vi "parse_tree.vi"() -> ()   [LabVIEW 2021]
uses:
  <vilib>/National Instruments/Tree Map/Tree Map.lvlib
panel:
  out "Pretty XML":string
  in  "Expression":string="(((1+2)*3)/(3+9))"
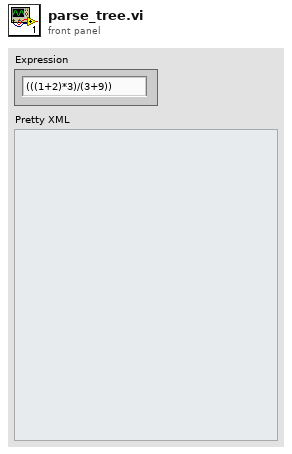
[diagram p1: front panel]
types:
  T1 = typedef "Tree Map.lvlib/Tree Map Data.ctl" = map{string, cluster{"Child Paths Set":set{string}, "Name":string, "Data":string, "Attributes":map{string, string}}}
  T2 = cluster{"Child Paths Set":set{string}, "Name":string, "Data":string, "Attributes":map{string, string}}
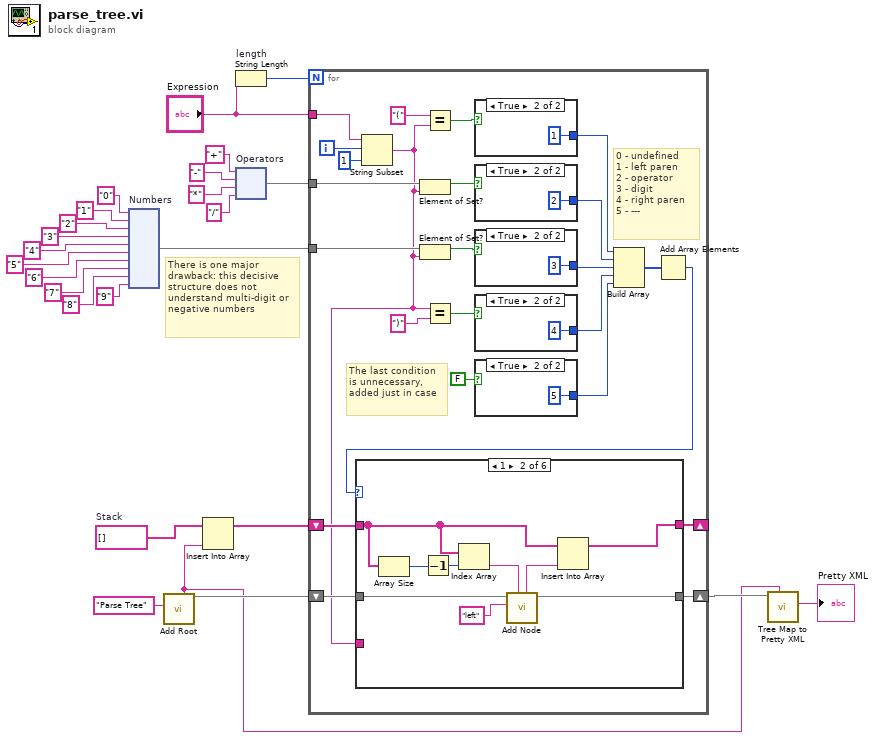
[diagram p0: block diagram]
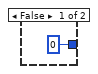
[diagram p2: hidden frame]
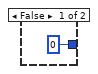
[diagram p3: hidden frame]
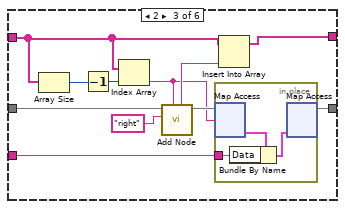
[diagram p5: hidden frame]
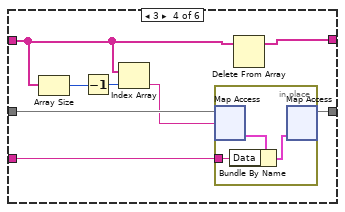
[diagram p6: hidden frame]
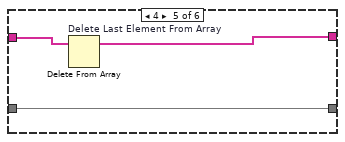
[diagram p7: hidden frame]
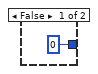
[diagram p9: hidden frame]
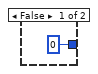
[diagram p10: hidden frame]
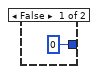
[diagram p11: hidden frame]
diagram:
  w6 = string[] []  # Stack
  # "There is one major drawback: this decisive structure does not understand multi-digit or negative numbers"
  n1 = node "Numbers"("0" ("element"), "1" ("element"), "2" ("element"), "3" ("element"), "4" ("element"), "5" ("element"), "6" ("element"), "7" ("element"), "8" ("element"), "9" ("element")) -> (w8:set{string})
  n2 = call <vilib>:"Add Root.vi"("New Root Name"="Parse Tree") -> ("Tree Map Out"=w3:T1, "Root Path"=w1:string)  [unwired: 9 in]
  n3 = Insert Into Array "Insert Into Array"(array=w6, new element=w1) -> (w5:string[])  [unwired: 1 in]
  n4 = String Length "length"(string="Expression") -> (length=w21:i32)
  n5 = node "Operators"("+" ("element"), "-" ("element"), "*" ("element"), "/" ("element")) -> (w9:set{string})
  n6 = for {
    N: w21 -> [_]
    tunnel: "Expression" -> [w49]
    tunnel: w9 -> [w45]
    tunnel: w8 -> [w43]
    shift-right: [w37] -> w2
    shift-left: w3 -> [w40]
    shift-right: [w38] -> _
    shift-left: w5 -> [w39]
    i -> [w48]
    # "The last condition is unnecessary, added just in case"
    # "0 - undefined\n1 - left paren\n2 - operator\n3 - digit\n4 - right paren\n5 - ---"
    n7 = String Subset(string=w49, offset (0)=w48, length (rest)=1 ("length (rest)")) -> (substring=w26:string)
    n8 = Element of Set?(10:w26, 11:w45) -> (3:w46:bool)
    n9 = Element of Set?(10:w26, 11:w43) -> (3:w44:bool)
    n10 = Equal?(x="(", y=w26) -> (x = y?=w30:bool)
    n11 = Equal?(x=w26, y=")" ("x")) -> (x = y?=w28:bool)
    n12 = case shown="True" w30 {
      tunnel: [0 1] -> w35
      frame False {
      }
      frame True {
      }
    }
    n13 = case shown="True" w46 {
      tunnel: [0 2] -> w32
      frame False {
      }
      frame True {
      }
    }
    n14 = case shown="True" w44 {
      tunnel: [0 3] -> w36
      frame False {
      }
      frame True {
      }
    }
    n15 = case shown="True" w28 {
      tunnel: [0 4] -> w33
      frame False {
      }
      frame True {
      }
    }
    n16 = case shown="True" FALSE {
      tunnel: [0 5] -> w34
      frame False {
      }
      frame True {
      }
    }
    n17 = Build Array(w35, w32, w36, w33, w34) -> (w42:i32[])
    n18 = Add Array Elements(numeric array=w42) -> (sum=w41:i32)
    n19 = case shown="1" w41 {
      tunnel: w40 -> [w54 w64 w72 w85 w92 w93]
      tunnel: w39 -> [w55 w59 w69 w80 w91 w94]
      tunnel: [w55 w61 w67 w79 w90 w94] -> w38
      tunnel: [w54 w60 w75 w86 w92 w93] -> w37
      tunnel: w26 -> [_ _ w65 w81 _ _]
      frame 0, Default {
      }
      frame 1 {
        n20 = Array Size(array=w59) -> (size(s)=w58:i32)
        n21 = Decrement(x=w58) -> (x-1=w57:i32)
        n22 = Index Array "Index Array"(array=w59, index=w57) -> (element=w62:string)
        n23 = call <vilib>:"Add Node.vi"("Parent Path"=w62, "New Node Name"="left", "Tree Map In"=w64) -> ("Tree Map Out"=w60:T1, "New Node Path"=w56:string)  [unwired: 6 in, 1 out]
        n24 = Insert Into Array "Insert Into Array"(array=w59, new element=w56) -> (w61:string[])  [unwired: 1 in]
      }
      frame 2 {
        n25 = Array Size(array=w69) -> (size(s)=w73:i32)
        n26 = Decrement(x=w73) -> (x-1=w74:i32)
        n27 = Index Array "Index Array"(array=w69, index=w74) -> (element=w66:string)
        n28 = call <vilib>:"Add Node.vi"("Parent Path"=w66, "New Node Name"="right", "Tree Map In"=w72) -> ("Tree Map Out"=w71:T1, "New Node Path"=w68:string)  [unwired: 6 in, 1 out]
        n29 = in-place {
          in-place-border: w65 -> [w76]
          n30 = in-place-map #1(w71, w66) -> (w77:T2)  [unwired: 1 in, 1 out]
          n31 = Bundle By Name(cluster=w77, "Data"=w76) -> (w78:T2)
          n32 = in-place-map #1(w78) -> (w75:T1)  [unwired: 1 in, 2 out]
        }
        n33 = Insert Into Array "Insert Into Array"(array=w69, new element=w68) -> (w67:string[])  [unwired: 1 in]
      }
      frame 3 {
        n34 = Array Size(array=w80) -> (size(s)=w83:i32)
        n35 = Decrement(x=w83) -> (x-1=w84:i32)
        n36 = Index Array "Index Array"(array=w80, index=w84) -> (element=w82:string)
        n37 = in-place {
          in-place-border: w81 -> [w87]
          n38 = in-place-map #2(w85, w82) -> (w88:T2)  [unwired: 1 in, 1 out]
          n39 = Bundle By Name(cluster=w88, "Data"=w87) -> (w89:T2)
          n40 = in-place-map #2(w89) -> (w86:T1)  [unwired: 1 in, 2 out]
        }
        n41 = Delete From Array "Delete From Array"(array=w80) -> (array with subset deleted=w79:string[])  [unwired: 2 in, 1 out]
      }
      frame 4 {
        n42 = Delete From Array "Delete Last Element From Array"(array=w91) -> (array with subset deleted=w90:string[])  [unwired: 2 in, 1 out]
      }
      frame 5 {
      }
    }
  }
  n43 = call <vilib>:"Tree Map to Pretty XML.vi"("Root Path"=w1, "Tree Map In"=w2) -> ("Pretty XML"=→"Pretty XML":string)  [unwired: 8 in, 1 out]
